vi "Create SuBUS Waveform.vi"(7 "sample rate":dbl=1000.0 format="%#_6p", 8 "error in (no error)":errorcluster, 9 "Reg_Address_Data":T2={"Address"=81, "Data"=0} {"Address" format="%.0x"}, 10 "USID":T1=13 max=15, 11 "OVS":u8=16) -> (0 "error out":errorcluster, 3 "Digital Waveform Graph":digitalwaveform(graph))   [LabVIEW 2013]
uses:
  Controls/Reg_Address_Data.ctl
  Controls/USID.ctl
  <vilib>/Waveform/DWDTOps.llb/DWDT Append Digital Samples.vi
  <vilib>/Waveform/DWDTOps.llb/Digital Pattern Generator (Single Value).vi
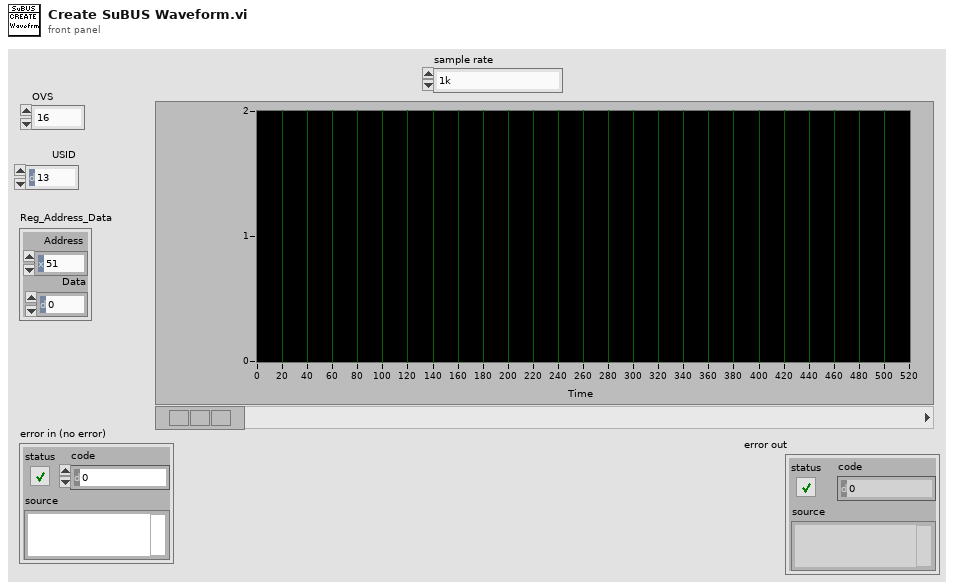
[diagram p1: front panel]
types:
  T1 = typedef "USID.ctl" = u8
  T2 = typedef "Reg_Address_Data.ctl" = cluster{"Address":u8, "Data":u8}
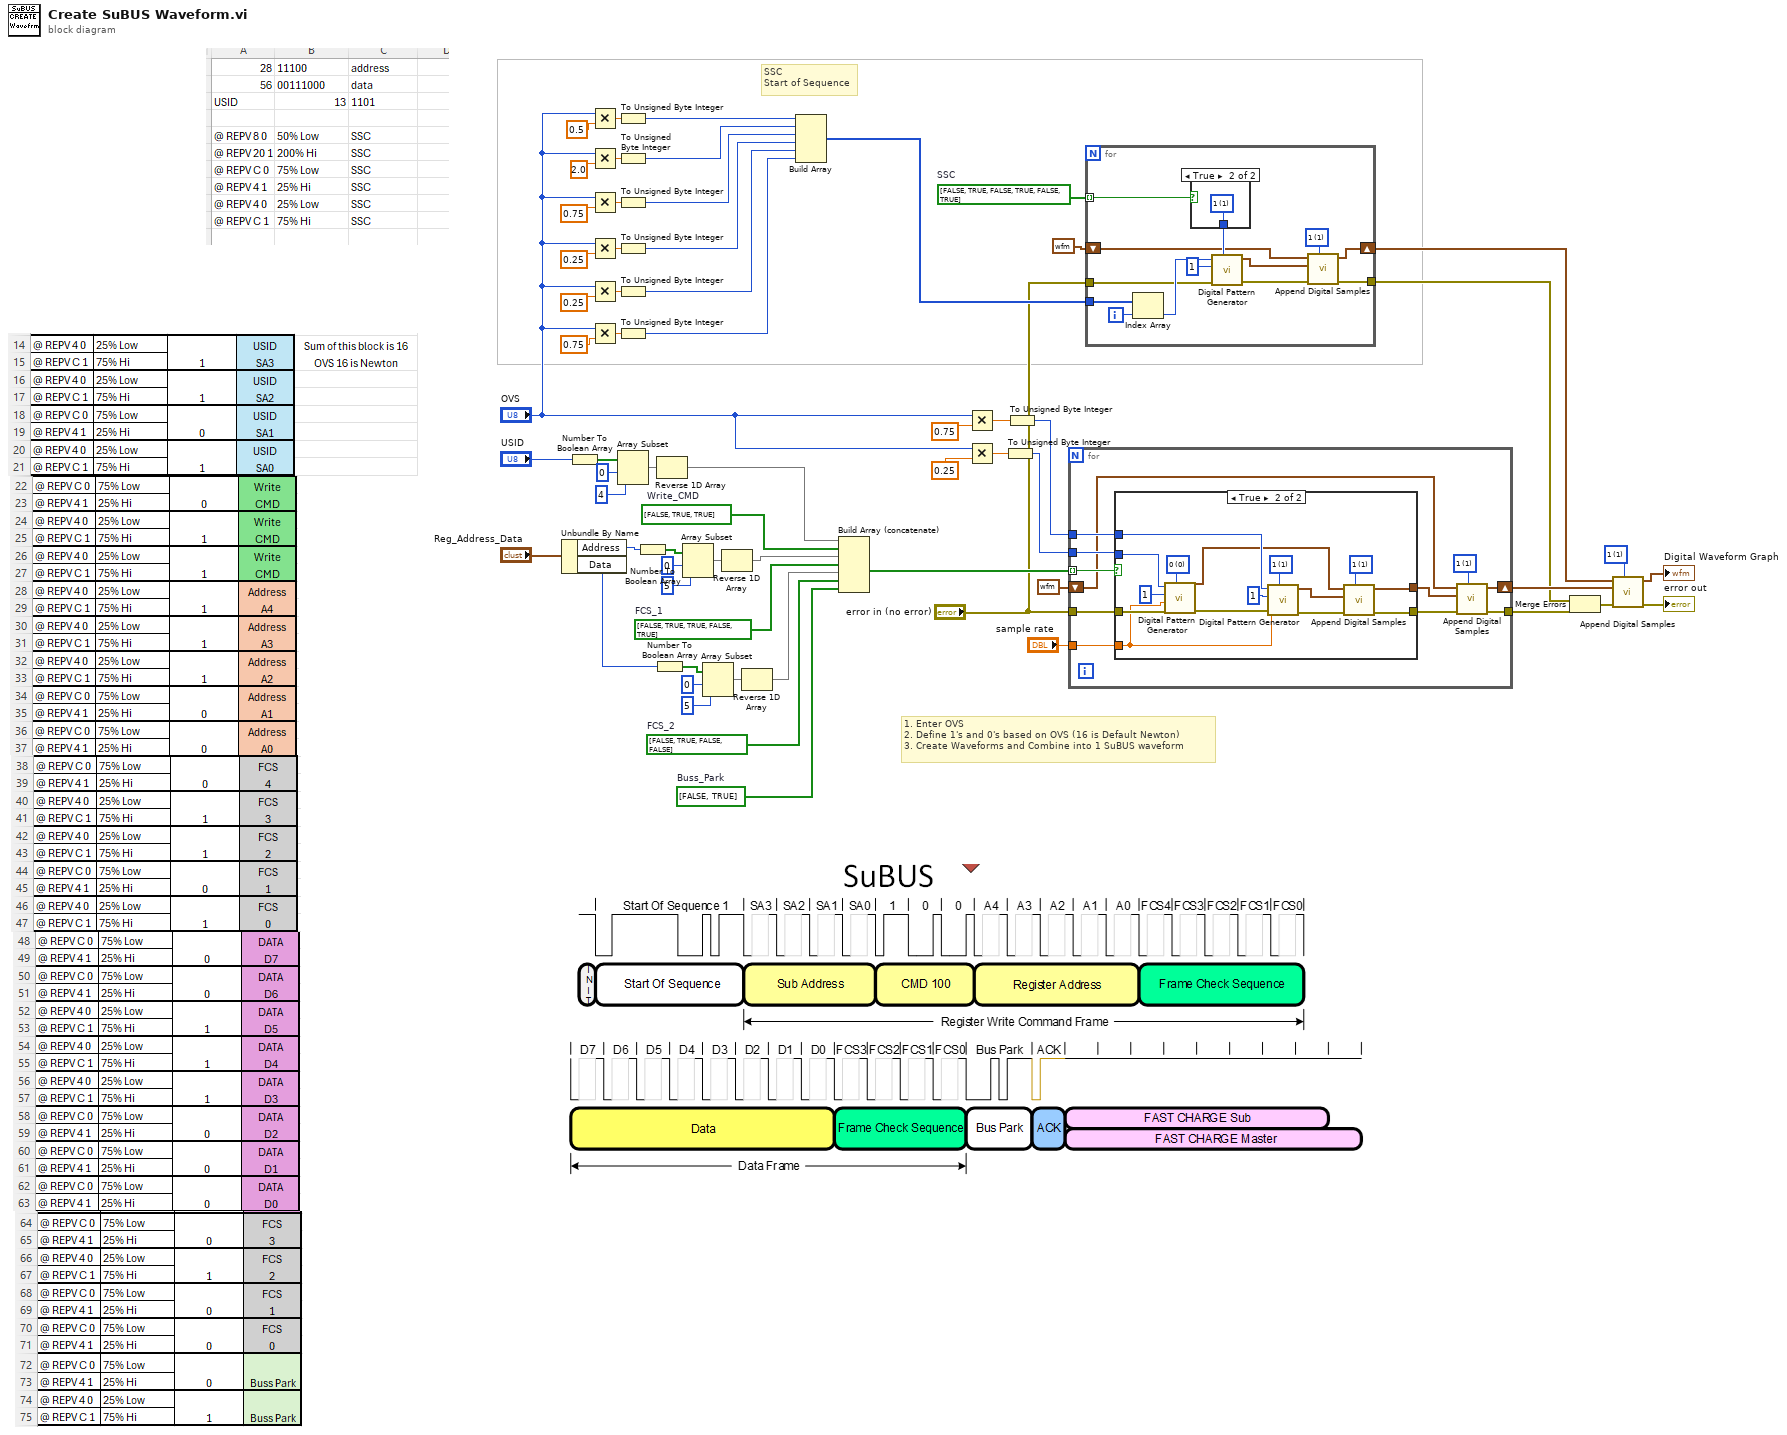
[diagram p0: block diagram]
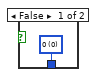
[diagram p2: hidden frame]
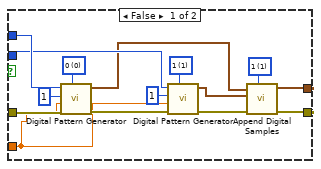
[diagram p3: hidden frame]
diagram:
  w7 = u8 1 items=["0", "1", "Z", "L", "H", "X", "T", "V"] ("default value")
  w11 = bool[] [FALSE, TRUE, FALSE, TRUE, FALSE, TRUE]  # SSC
  w34 = bool[] [FALSE, TRUE]  # Buss_Park
  w35 = bool[] [FALSE, TRUE, FALSE, FALSE]  # FCS_2
  w43 = bool[] [FALSE, TRUE, TRUE, FALSE, TRUE]  # FCS_1
  w50 = bool[] [FALSE, TRUE, TRUE]  # Write_CMD
  # "SSC\nStart of Sequence"
  # "1. Enter OVS\n2. Define 1's and 0's based on OVS (16 is Default Newton)\n3. Create Waveforms and Combine into 1 SuBUS waveform"
  n1 = Unbundle By Name("Reg_Address_Data") -> ("Address"=w45:u8, "Data"=w37:u8)
  n2 = Number To Boolean Array(number="USID") -> (Boolean array=w59:bool[])
  n3 = Multiply(x="OVS", y=0.5) -> (x*y=w33:dbl)
  n4 = Multiply(x="OVS", y=2.0) -> (x*y=w31:dbl)
  n5 = Multiply(x="OVS", y=0.75) -> (x*y=w29:dbl)
  n6 = Multiply(x="OVS", y=0.25) -> (x*y=w27:dbl)
  n7 = Multiply(x="OVS", y=0.25) -> (x*y=w25:dbl)
  n8 = Multiply(x="OVS", y=0.75) -> (x*y=w23:dbl)
  n9 = To Unsigned Byte Integer(number=w33) -> (unsigned 8bit integer=w18:u8)
  n10 = To Unsigned Byte Integer(number=w31) -> (unsigned 8bit integer=w17:u8)
  n11 = To Unsigned Byte Integer(number=w29) -> (unsigned 8bit integer=w16:u8)
  n12 = To Unsigned Byte Integer(number=w27) -> (unsigned 8bit integer=w15:u8)
  n13 = To Unsigned Byte Integer(number=w25) -> (unsigned 8bit integer=w14:u8)
  n14 = To Unsigned Byte Integer(number=w23) -> (unsigned 8bit integer=w13:u8)
  n15 = Array Subset(array=w59, index=0, length=4) -> (w58:bool[])
  n16 = Number To Boolean Array(number=w45) -> (Boolean array=w47:bool[])
  n17 = Number To Boolean Array(number=w37) -> (Boolean array=w39:bool[])
  n18 = Reverse 1D Array(array=w58) -> (reversed array=w51:bool[])
  n19 = Array Subset(array=w47, index=0, length=5) -> (w46:bool[])
  n20 = Array Subset(array=w39, index=0, length=5) -> (w38:bool[])
  n21 = Reverse 1D Array(array=w46) -> (reversed array=w44:bool[])
  n22 = Reverse 1D Array(array=w38) -> (reversed array=w36:bool[])
  n23 = Build Array(w18, w17, w16, w15, w14, w13) -> (w12:u8[])
  n24 = Build Array (concatenate)(w51, w50, w44, w43, w36, w35, w34) -> (w42:bool[])
  n25 = Multiply(x="OVS", y=0.75) -> (x*y=w55:dbl)
  n26 = Multiply(x="OVS", y=0.25) -> (x*y=w54:dbl)
  n27 = To Unsigned Byte Integer(number=w54) -> (unsigned 8bit integer=w52:u8)
  n28 = To Unsigned Byte Integer(number=w55) -> (unsigned 8bit integer=w53:u8)
  n29 = for {
    tunnel: w42 -> [w72] mode=indexing
    tunnel: w53 -> [w74]
    tunnel: w52 -> [w73]
    shift-right: [w69] -> w8
    shift-left: digitalwaveform {"t0"=timestamp(0 s since 1904-01-01), "dt"=0.0, "Y"={"transitions"=[], "data"=[]}} ("digital waveform out") -> [w65]
    tunnel: "error in (no error)" -> [w67]
    tunnel: [w66] -> w3
    tunnel: "sample rate" -> [w64]
    w68 = u8 1 items=["0", "1", "Z", "L", "H", "X", "T", "V"] ("default value")
    n30 = case shown="True" w72 {
      tunnel: w74 -> [w87 w98]
      tunnel: w73 -> [w82 w99]
      tunnel: [w79 w94] -> w70
      tunnel: [w78 w93] -> w71
      tunnel: w67 -> [w76 w91]
      tunnel: w64 -> [w75 w90]
      frame False {
        w77 = u8 1 items=["0", "1", "Z", "L", "H", "X", "T", "V"] ("default value")
        w85 = u8 1 items=["0", "1", "Z", "L", "H", "X", "T", "V"] ("value")
        w88 = u8 0 items=["0", "1", "Z", "L", "H", "X", "T", "V"] ("value")
        n31 = call-poly <vilib>:"Digital Pattern Generator.vi"("value"=w88, "error in (no error)"=w76, "sample rate"=w75, "number of signals"=u32 1, "number of samples"=w87) -> ("error out"=w84:errorcluster, "digital waveform"=w81:digitalwaveform)  [unwired: 5 in]
        n32 = call-poly <vilib>:"Digital Pattern Generator.vi"("value"=w85, "error in (no error)"=w84, "sample rate"=w75, "number of signals"=u32 1, "number of samples"=w82) -> ("error out"=w83:errorcluster, "digital waveform"=w80:digitalwaveform)  [unwired: 5 in]
        n33 = call-poly <vilib>:"Append Digital Samples.vi"("default value"=w77, "error in (no error)"=w83, "digital waveform B"=w80, "digital waveform A"=w81) -> ("error out"=w78:errorcluster, "digital waveform out"=w79:digitalwaveform)  [unwired: 6 in]
      }
      frame True {
        w92 = u8 1 items=["0", "1", "Z", "L", "H", "X", "T", "V"] ("default value")
        w101 = u8 1 items=["0", "1", "Z", "L", "H", "X", "T", "V"] ("value")
        w104 = u8 0 items=["0", "1", "Z", "L", "H", "X", "T", "V"] ("value")
        n34 = call-poly <vilib>:"Digital Pattern Generator.vi"("value"=w104, "error in (no error)"=w91, "sample rate"=w90, "number of signals"=u32 1, "number of samples"=w99) -> ("error out"=w97:errorcluster, "digital waveform"=w96:digitalwaveform)  [unwired: 5 in]
        n35 = call-poly <vilib>:"Digital Pattern Generator.vi"("value"=w101, "error in (no error)"=w97, "sample rate"=w90, "number of signals"=u32 1, "number of samples"=w98) -> ("error out"=w100:errorcluster, "digital waveform"=w95:digitalwaveform)  [unwired: 5 in]
        n36 = call-poly <vilib>:"Append Digital Samples.vi"("default value"=w92, "error in (no error)"=w100, "digital waveform B"=w95, "digital waveform A"=w96) -> ("error out"=w93:errorcluster, "digital waveform out"=w94:digitalwaveform)  [unwired: 6 in]
      }
    }
    n37 = call-poly <vilib>:"Append Digital Samples.vi"("default value"=w68, "error in (no error)"=w71, "digital waveform B"=w70, "digital waveform A"=w65) -> ("error out"=w66:errorcluster, "digital waveform out"=w69:digitalwaveform)  [unwired: 6 in]
  }
  n38 = for {
    tunnel: w12 -> [w117]
    tunnel: w11 -> [w114] mode=indexing
    shift-right: [w108] -> w9
    shift-left: digitalwaveform {"t0"=timestamp(0 s since 1904-01-01), "dt"=0.0, "Y"={"transitions"=[], "data"=[]}} ("digital waveform out") -> [w107]
    tunnel: "error in (no error)" -> [w106]
    tunnel: [w105] -> w4
    i -> [w116]
    w111 = u8 1 items=["0", "1", "Z", "L", "H", "X", "T", "V"] ("default value")
    n39 = Index Array(array=w117, index=w116) -> (element=w112:u8)
    n40 = case shown="True" w114 {
      tunnel: [w118 w119] -> w113
      frame False {
        w118 = u8 0 items=["0", "1", "Z", "L", "H", "X", "T", "V"] ("value")
      }
      frame True {
        w119 = u8 1 items=["0", "1", "Z", "L", "H", "X", "T", "V"] ("value")
      }
    }
    n41 = call-poly <vilib>:"Digital Pattern Generator.vi"("value"=w113, "error in (no error)"=w106, "number of signals"=u32 1, "number of samples"=w112) -> ("error out"=w110:errorcluster, "digital waveform"=w109:digitalwaveform)  [unwired: 6 in]
    n42 = call-poly <vilib>:"Append Digital Samples.vi"("default value"=w111, "error in (no error)"=w110, "digital waveform B"=w109, "digital waveform A"=w107) -> ("error out"=w105:errorcluster, "digital waveform out"=w108:digitalwaveform)  [unwired: 6 in]
  }
  n43 = Merge Errors(w4, w3) -> (w2:errorcluster)
  n44 = call-poly <vilib>:"Append Digital Samples.vi"("default value"=w7, "error in (no error)"=w2, "digital waveform B"=w8, "digital waveform A"=w9) -> ("error out"=→"error out":errorcluster, "digital waveform out"=→"Digital Waveform Graph":digitalwaveform)  [unwired: 6 in]
